vi "FTW-DevUtil-ClassGenealogyWipe.vi"() -> ()   [LabVIEW 2013]
uses:
  System.Xml
panel:
  out "error out":errorcluster
  out "Results":string[][](table)
  in  "Folder to Search for Classes":path
  # "Be sure to have everything committed before running this tool so you can revert if needed"
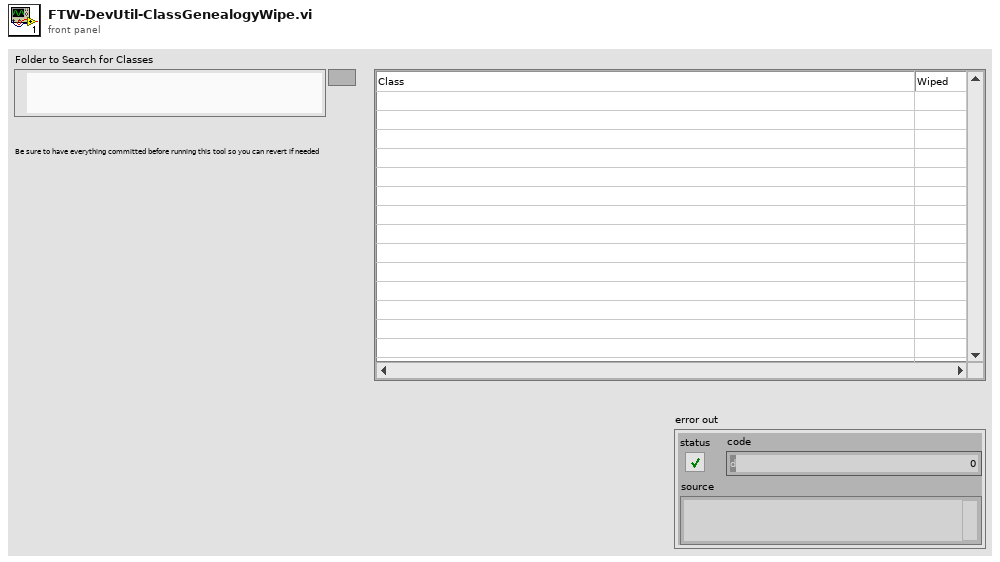
[diagram p1: front panel]
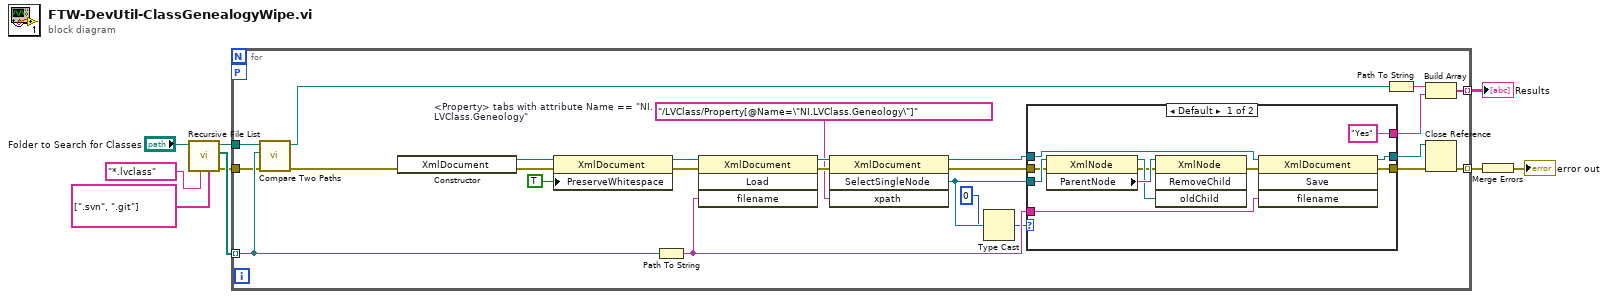
[diagram p0: block diagram]
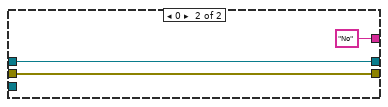
[diagram p2: hidden frame]
diagram:
  n1 = call <vilib>:"Recursive File List.vi"("Folders to Exclude"=string[] [".svn", ".git"], "pattern"="*.lvclass", "Folder Path"="Folder to Search for Classes") -> ("error out"=w7:errorcluster, "All Files in Dir"=w8:path[], "dup Folder Path"=w1:path)  [unwired: 4 in, 2 out]
  n2 = for {
    tunnel: w8 -> [w29] mode=indexing
    tunnel: w7 -> [w11]
    tunnel: [w21] -> w6 mode=indexing
    tunnel: [w34] -> w4 mode=indexing
    tunnel: w1 -> [w33]
    workers-P: _ -> [_]
    w26 = "/LVClass/Property[@Name=\"NI.LVClass.Geneology\"]"  # <Property> tabs with attribute Name == "NI.LVClass.Geneology"
    n3 = call <vilib>:"Compare Two Paths.vi"("error in (no error)"=w11, "Path 2"=w29, "Path 1"=w33) -> ("error out"=w10:errorcluster, "Relative Path from 1 to 2"=w32:path)  [unwired: 5 in, 2 out]
    n4 = constructor class="XmlDocument"(error in=w10) -> (reference out=w14:refnum<k24>, error out=w30:errorcluster)  [unwired: 2 in, 1 out]
    n5 = property class="XmlDocument"(reference=w14, error in=w30, "PreserveWhitespace"=TRUE) -> (reference out=w13:refnum<k24>, error out=w15:errorcluster)
    n6 = Path To String(path=w29) -> (string=w24:string)
    n7 = invoke class="XmlDocument" method="Load"(reference=w13, error in=w15, "filename"=w24) -> (reference out=w28:refnum<k24>, error out=w27:errorcluster)  [unwired: 1 in, 2 out]
    n8 = invoke class="XmlDocument" method="SelectSingleNode"(reference=w28, error in=w27, "xpath"=w26) -> (reference out=w25:refnum<k24>, error out=w19:errorcluster, "SelectSingleNode"=w18:refnum<k24>)  [unwired: 1 in, 1 out]
    n9 = Type Cast(type=0, x=w18) -> (*(type *) &x=w16:i32)
    n10 = case shown="Default" w16 {
      tunnel: w18 -> [w45 _]
      tunnel: w25 -> [w41 w48]
      tunnel: w24 -> [w35 _]
      tunnel: [w37 w46] -> w23
      tunnel: [w40 w48] -> w22
      tunnel: ["Yes" ("XPath expression") "No" ("XPath expression")] -> w20
      tunnel: w19 -> [w38 w46]
      frame Default {
        n11 = property class="XmlNode"(reference=w45, error in=w38) -> (reference out=w43:refnum<k24>, error out=w42:errorcluster, "ParentNode"=w44:refnum<k24>)
        n12 = invoke class="XmlNode" method="RemoveChild"(reference=w44, error in=w42, "oldChild"=w43) -> (error out=w36:errorcluster)  [unwired: 1 in, 3 out]
        n13 = invoke class="XmlDocument" method="Save"(reference=w41, error in=w36, "filename"=w35) -> (reference out=w40:refnum<k24>, error out=w37:errorcluster)  [unwired: 1 in, 2 out]
      }
      frame 0 {
      }
    }
    n14 = Path To String(path=w32) -> (string=w31:string)
    n15 = Build Array(w31, w20) -> (w34:string[])
    n16 = Close Reference(reference=w22, error in (no error)=w23) -> (error out=w21:errorcluster)
  }
  "Results" <- w4
  n17 = Merge Errors(w6) -> (→"error out":errorcluster)
